vi "201641053020卢泽烽.vi"() -> ()   [LabVIEW 2017]
uses:
  <vilib>/measure/NI_MABase.lvlib
  <vilib>/measure/NI_MAPro.lvlib
panel:
  in  "频率":dbl=10.0 format="%0.2p"
  in  "停止":bool
  in  "信噪比":dbl
  in  "公式":string="sin(w*t)*sin(2*pi(1)*t)"
  in  "方波占空比":dbl=50.0 caption="占空比(%)" format="%0.2f"
  in  "采样信息":cluster{"Fs":dbl, "#s":dbl}={"Fs"=1000.0, "#s"=1000.0} {"Fs" format="%.2p"}
  in  "相位":dbl format="%.2p"
  in  "幅值":dbl=1.0 format="%0.2p"
  in  "波形选择":enum16{"公式波", "三角波", "方波", "正弦波"}(ring)
  in  "噪声选择":enum16{"均匀白噪声", "高斯白噪声", "无"}(ring)
  out "波形图":waveform(dbl)(graph)
  # "波形发生器"
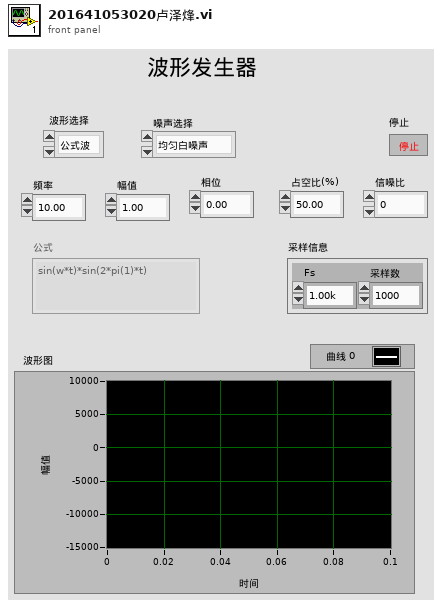
[diagram p1: front panel]
types:
  T1 = enum8{"Enabled", "Disabled", "Disabled and Grayed Out"}
  T2 = enum16{"Sine Wave", "Triangle Wave", "Square Wave", "Sawtooth Wave"}
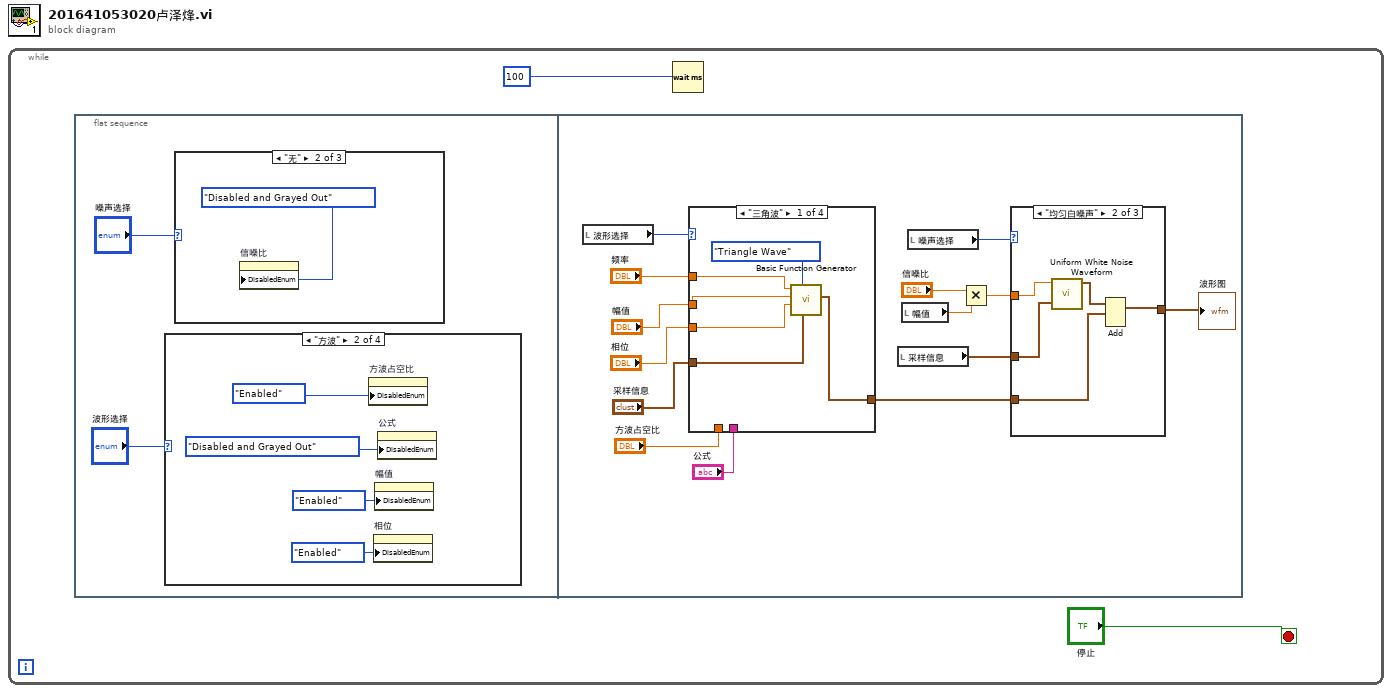
[diagram p0: block diagram]
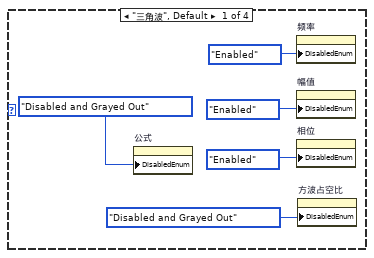
[diagram p2: hidden frame]
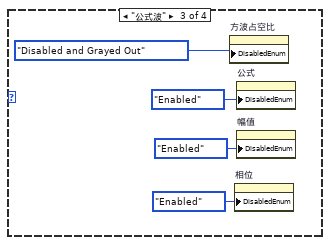
[diagram p3: hidden frame]
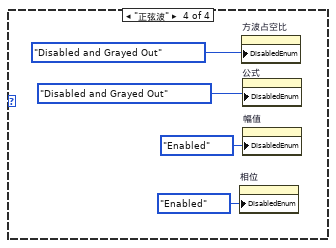
[diagram p4: hidden frame]
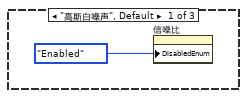
[diagram p5: hidden frame]
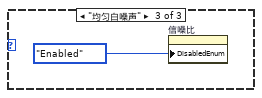
[diagram p6: hidden frame]
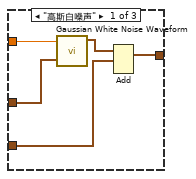
[diagram p7: hidden frame]
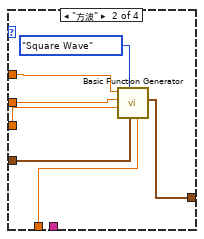
[diagram p9: hidden frame]
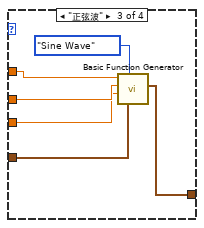
[diagram p10: hidden frame]
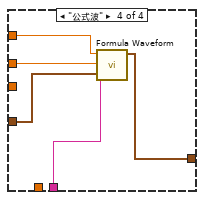
[diagram p11: hidden frame]
diagram:
  n1 = while {
    stop <- "停止" stop-if-true
    n2 = flat-sequence {
      frame #0 {
        n3 = case shown="\"方波\"" "波形选择" {
          frame "三角波", Default {
            n4 = property on="公式" class="Str"("DisabledEnum"=T1."Disabled and Grayed Out" ("禁用")) -> ()  [unwired: 2 in, 2 out]
            n5 = property on="频率" class="DigNum (严格)"("DisabledEnum"=T1."Enabled" ("禁用")) -> ()  [unwired: 2 in, 2 out]
            n6 = property on="幅值" class="DigNum (严格)"("DisabledEnum"=T1."Enabled" ("禁用")) -> ()  [unwired: 2 in, 2 out]
            n7 = property on="相位" class="DigNum (严格)"("DisabledEnum"=T1."Enabled" ("禁用")) -> ()  [unwired: 2 in, 2 out]
            n8 = property on="方波占空比" class="DigNum (严格)"("DisabledEnum"=T1."Disabled and Grayed Out" ("禁用")) -> ()  [unwired: 2 in, 2 out]
          }
          frame "方波" {
            n9 = property on="方波占空比" class="DigNum (严格)"("DisabledEnum"=T1."Enabled" ("禁用")) -> ()  [unwired: 2 in, 2 out]
            n10 = property on="相位" class="DigNum (严格)"("DisabledEnum"=T1."Enabled" ("禁用")) -> ()  [unwired: 2 in, 2 out]
            n11 = property on="幅值" class="DigNum (严格)"("DisabledEnum"=T1."Enabled" ("禁用")) -> ()  [unwired: 2 in, 2 out]
            n12 = property on="公式" class="Str"("DisabledEnum"=T1."Disabled and Grayed Out" ("禁用")) -> ()  [unwired: 2 in, 2 out]
          }
          frame "公式波" {
            n13 = property on="方波占空比" class="DigNum (严格)"("DisabledEnum"=T1."Disabled and Grayed Out" ("禁用")) -> ()  [unwired: 2 in, 2 out]
            n14 = property on="相位" class="DigNum (严格)"("DisabledEnum"=T1."Enabled" ("禁用")) -> ()  [unwired: 2 in, 2 out]
            n15 = property on="公式" class="Str"("DisabledEnum"=T1."Enabled" ("禁用")) -> ()  [unwired: 2 in, 2 out]
            n16 = property on="幅值" class="DigNum (严格)"("DisabledEnum"=T1."Enabled" ("禁用")) -> ()  [unwired: 2 in, 2 out]
          }
          frame "正弦波" {
            n17 = property on="相位" class="DigNum (严格)"("DisabledEnum"=T1."Enabled" ("禁用")) -> ()  [unwired: 2 in, 2 out]
            n18 = property on="方波占空比" class="DigNum (严格)"("DisabledEnum"=T1."Disabled and Grayed Out" ("禁用")) -> ()  [unwired: 2 in, 2 out]
            n19 = property on="公式" class="Str"("DisabledEnum"=T1."Disabled and Grayed Out" ("禁用")) -> ()  [unwired: 2 in, 2 out]
            n20 = property on="幅值" class="DigNum (严格)"("DisabledEnum"=T1."Enabled" ("禁用")) -> ()  [unwired: 2 in, 2 out]
          }
        }
        n21 = case shown="\"无\"" "噪声选择" {
          frame "高斯白噪声", Default {
            n22 = property on="信噪比" class="DigNum (严格)"("DisabledEnum"=T1."Enabled" ("禁用")) -> ()  [unwired: 2 in, 2 out]
          }
          frame "无" {
            n23 = property on="信噪比" class="DigNum (严格)"("DisabledEnum"=T1."Disabled and Grayed Out" ("禁用")) -> ()  [unwired: 2 in, 2 out]
          }
          frame "均匀白噪声" {
            n24 = property on="信噪比" class="DigNum (严格)"("DisabledEnum"=T1."Enabled" ("禁用")) -> ()  [unwired: 2 in, 2 out]
          }
        }
      }
      frame #1 {
        n25 = local read "波形选择"() -> (w38:enum16{"公式波", "三角波", "方波", "正弦波"})
        n26 = case shown="\"三角波\"" w38 {
          tunnel: "幅值" -> [w54 w61 w67 w73]
          tunnel: "相位" -> [w53 w60 w66 _]
          tunnel: "采样信息" -> [w52 w59 w65 w72]
          tunnel: "方波占空比" -> [_ w58 _ _]
          tunnel: "公式" -> [_ _ _ w71]
          tunnel: [w51 w57 w64 w70] -> w27
          tunnel: "频率" -> [w50 w56 w63 w69]
          frame "三角波" {
            n27 = call <vilib>:"Basic Function Generator.vi"("sampling info"=w52, "signal type"=T2."Triangle Wave", "phase"=w53, "amplitude"=w54, "frequency"=w50) -> ("signal out"=w51:waveform(dbl))  [unwired: 4 in, 2 out]
          }
          frame "方波" {
            n28 = call <vilib>:"Basic Function Generator.vi"("square wave duty cycle (%)"=w58, "sampling info"=w59, "signal type"=T2."Square Wave", "phase"=w60, "amplitude"=w61, "frequency"=w56) -> ("signal out"=w57:waveform(dbl))  [unwired: 3 in, 2 out]
          }
          frame "正弦波" {
            n29 = call <vilib>:"Basic Function Generator.vi"("sampling info"=w65, "signal type"=T2."Sine Wave", "phase"=w66, "amplitude"=w67, "frequency"=w63) -> ("signal out"=w64:waveform(dbl))  [unwired: 4 in, 2 out]
          }
          frame "公式波" {
            n30 = call <vilib>:"Formula Waveform.vi"("sampling info"=w72, "formula"=w71, "amplitude"=w73, "frequency"=w69) -> ("signal out"=w70:waveform(dbl))  [unwired: 6 in, 1 out]
          }
        }
        n31 = local read "采样信息"() -> (w28:cluster{"Fs":dbl, "#s":dbl})
        n32 = local read "幅值"() -> (w30:dbl)
        n33 = local read "噪声选择"() -> (w37:enum16{"均匀白噪声", "高斯白噪声", "无"})
        n34 = Multiply(x="信噪比", y=w30) -> (x*y=w29:dbl)
        n35 = case shown="\"均匀白噪声\"" w37 {
          tunnel: w29 -> [w43 w48 _]
          tunnel: w28 -> [w42 w47 _]
          tunnel: w27 -> [w41 w44 w49]
          tunnel: [w39 w45 w49] -> w26
          frame "高斯白噪声" {
            n36 = call <vilib>:"Gaussian White Noise Waveform.vi"("sampling info"=w42, "standard deviation"=w43) -> ("signal out"=w40:waveform(dbl))  [unwired: 8 in, 1 out]
            n37 = Add(1:w41, 2:w40) -> (0:w39:waveform(dbl))  [unwired: 1 in, 1 out]
          }
          frame "均匀白噪声" {
            n38 = call <vilib>:"Uniform White Noise Waveform.vi"("sampling info"=w47, "amplitude"=w48) -> ("signal out"=w46:waveform(dbl))  [unwired: 8 in, 1 out]
            n39 = Add(1:w44, 2:w46) -> (0:w45:waveform(dbl))  [unwired: 1 in, 1 out]
          }
          frame "无" {
          }
        }
        "波形图" <- w26
      }
    }
    n40 = Wait (ms)(milliseconds to wait=u32 100 ("等待时间（毫秒）")) -> ()  [unwired: 1 out]
  }
